vi "set and get ring values.vi"(7 "function":enum16{"Set", "Get"}(ring), 8 "error in (no error)":errorcluster, 10 "user options":T1, 11 "Ring Ref":refnum<vi>[](array[refnum])) -> (0 "error out":errorcluster, 2 "values & indexes":string[](array[string]))   [LabVIEW 2024]
uses:
  controls/ring data.ctl
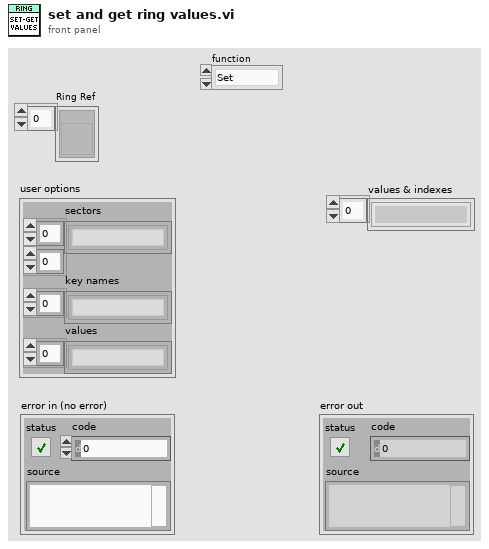
[diagram p1: front panel]
types:
  T1 = typedef "ring data.ctl" = cluster{"sectors":string[][], "key names":string[], "values":string[]}
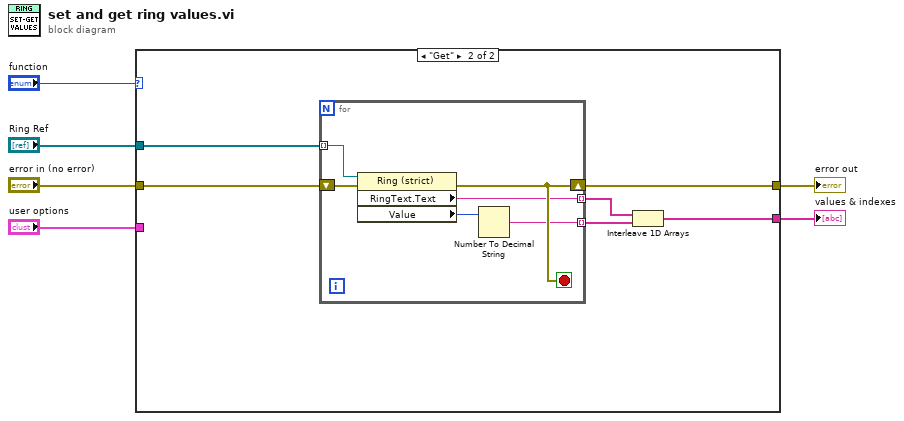
[diagram p0: block diagram]
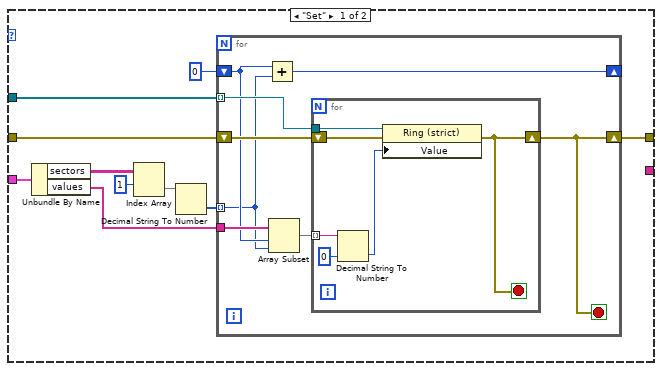
[diagram p2: hidden frame]
diagram:
  n1 = case shown="\"Get\"" "function" {
    tunnel: [w16 w32] -> w6
    tunnel: "error in (no error)" -> [w11 w33]
    tunnel: "Ring Ref" -> [w10 w34]
    tunnel: "user options" -> [w9 _]
    tunnel: [_ w31] -> w2
    frame "Set" {
      n2 = Unbundle By Name(w9) -> ("sectors"=w8:string[][], "values"=w7:string[])
      n3 = Index Array(array=w8, index (row)=1) -> (element=w13:string[])  [unwired: 1 in]
      n4 = Decimal String To Number(string=w13) -> (number=w14:i32[])  [unwired: 2 in, 1 out]
      n5 = for {
        tunnel: w10 -> [w24] mode=indexing
        shift-right: [w22] -> w16
        shift-left: w11 -> [w23]
        tunnel: w14 -> [w18] mode=indexing
        tunnel: w7 -> [w20]
        shift-right: [w21] -> _
        shift-left: 0 -> [w19]
        stop <- w22 stop-if-true
        n6 = Add(x=w19, y=w18) -> (x+y=w21:i32)
        n7 = Array Subset(array=w20, index=w19, length=w18) -> (w17:string[])
        n8 = for {
          tunnel: w24 -> [w30]
          tunnel: w17 -> [w28] mode=indexing
          shift-right: [w25] -> w22
          shift-left: w23 -> [w29]
          stop <- w25 stop-if-true
          n9 = Decimal String To Number(string=w28, default (0L)=u16 0 ("default (0 I32)")) -> (number=w26:u16)  [unwired: 1 in, 1 out]
          n10 = property on="Property Node" class="Ring (strict)"(reference=w30, error in=w29, "Value"=w26) -> (error out=w25:errorcluster)  [unwired: 1 out]
        }
      }
    }
    frame "Get" {
      n11 = for {
        tunnel: w34 -> [w41] mode=indexing
        tunnel: [w39] -> w35 mode=indexing
        tunnel: [w38] -> w36 mode=indexing
        shift-right: [w42] -> w32
        shift-left: w33 -> [w37]
        stop <- w42 stop-if-true
        n12 = property class="Ring (strict)"(reference=w41, error in=w37) -> (error out=w42:errorcluster, "RingText.Text"=w39:string, "Value"=w40:u16)  [unwired: 1 out]
        n13 = Number To Decimal String(number=w40) -> (decimal integer string=w38:string)  [unwired: 1 in]
      }
      n14 = Interleave 1D Arrays(w35, w36) -> (w31:string[])
    }
  }
  "error out" <- w6
  "values & indexes" <- w2
